vi "Write in Paquetes.vi"(8 "error in (no error)":errorcluster, 11 "TestCase in":refnum<class "Test DataBase.lvclass">) -> (0 "error out":errorcluster, 3 "TestCase out":refnum<class "Test DataBase.lvclass">)   [LabVIEW 2020, in "Test DataBase.lvclass"]
uses:
  Test DataBase.lvclass
  Paquetes Disponibles/Paquetes Disponibles.lvclass
  Paquetes Disponibles/Paquetes Disponibles.lvclass/Paquetes Disponibles.ctl
  <vilib>/addons/_JKI Toolkits/VI Tester/TestCase.llb/TestCase.lvclass
  C:/Program Files (x86)/National Instruments/LabVIEW 2020/vi.lib/addons/_JKI Toolkits/VI Tester/TestCase.llb/TestCase.lvclass
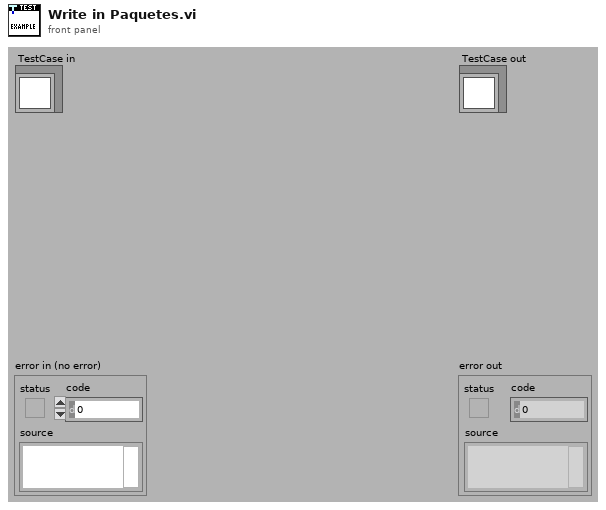
[diagram p1: front panel]
types:
  T1 = cluster{"Name":string, "Cost":u8, "Comprar":bool}[][]
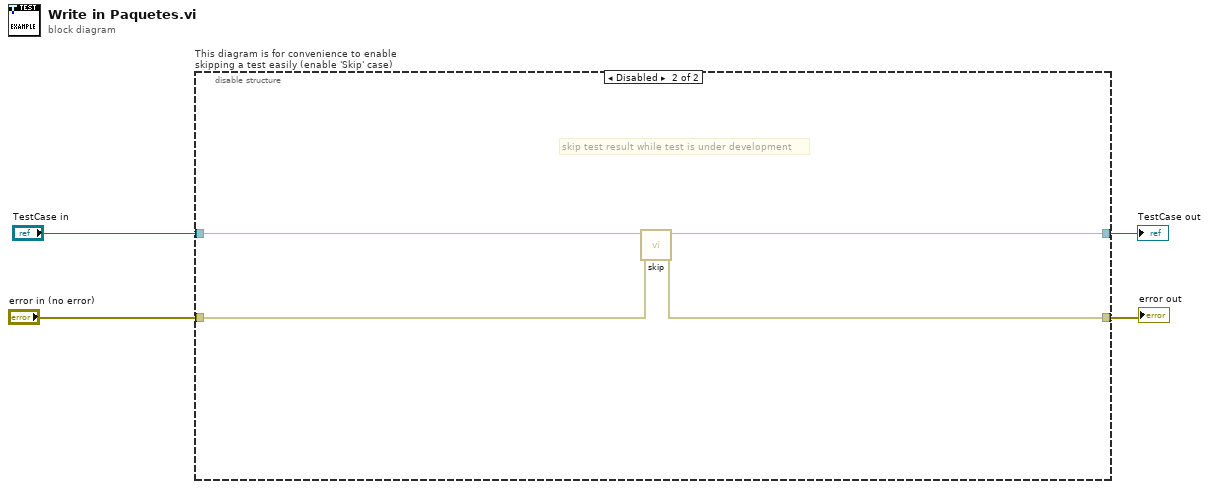
[diagram p0: block diagram]
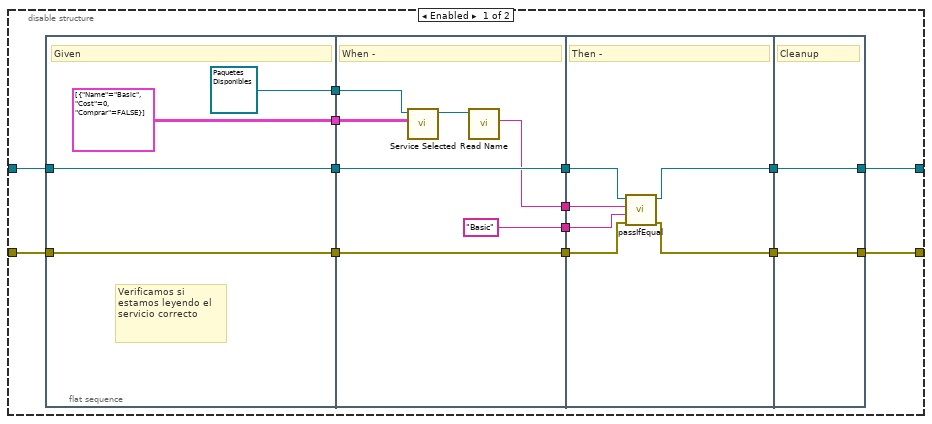
[diagram p2: hidden frame]
diagram:
  n1 = disable-structure "This diagram is for convenience to enable skipping a test easily (enable 'Skip' case)" shown="Disabled" {
    disable-tunnel: "TestCase in" -> [w12 w41]
    disable-tunnel: [w10 w39] -> w1
    disable-tunnel: [w9 w40] -> w3
    disable-tunnel: "error in (no error)" -> [w11 w38]
    frame Enabled {
      n2 = flat-sequence {
        tunnel: w11 -> [w21]
        tunnel: w12 -> [w22]
        tunnel: [w22] -> w18
        tunnel: [w21] -> w17
        tunnel: [refnum<class "Paquetes Disponibles.lvclass"> refnum ("Paquetes Disponibles.lvlib:Paquetes Disponibles.lvclass")] -> w8
        tunnel: [T1 [[{"Name"="Basic", "Cost"=0, "Comprar"=FALSE}]] ("Wash Car Cost")] -> w7
        tunnel: [w29] -> w16
        tunnel: [w28] -> w15
        tunnel: w18 -> [w29]
        tunnel: w17 -> [w28]
        tunnel: w8 -> [w27]
        tunnel: w7 -> [w26]
        tunnel: [w24] -> w6
        tunnel: ["Basic"] -> w5
        tunnel: [w34] -> w14
        tunnel: [w32] -> w13
        tunnel: w16 -> [w35]
        tunnel: w15 -> [w33]
        tunnel: w6 -> [w31]
        tunnel: w5 -> [w30]
        tunnel: [w36] -> w9
        tunnel: [w37] -> w10
        tunnel: w14 -> [w37]
        tunnel: w13 -> [w36]
        frame #0 {
          # "Verificamos si estamos leyendo el servicio correcto"
          # "Given"
        }
        frame #1 {
          # "When -"
          n3 = call "Service Selected.vi"("Wash Car Cost"=w26, "Paquetes Disponibles in"=w27) -> ("Paquetes Disponibles out"=w25:refnum<class "Paquetes Disponibles.lvclass">)  [unwired: 8 in, 1 out]
          n4 = call "Read Name.vi"("Paquetes Disponibles in"=w25) -> ("Name"=w24:string)  [unwired: 8 in, 2 out]
        }
        frame #2 {
          # "Then -"
          n5 = call-dynamic "passIfEqual.vi"("error in (no error)"=w33, "y"=w30, "x"=w31, "TestCase in"=w35) -> ("error out"=w32:errorcluster, "TestCase out"=w34:refnum<class "Test DataBase.lvclass">)  [unwired: 6 in]
        }
        frame #3 {
          # "Cleanup"
        }
      }
    }
    frame Disabled {
      # "skip test result while test is under development"
      n6 = call <vilib>:"skip.vi"("error in (no error)"=w38, "TestCase in"=w41) -> ("error out"=w40:errorcluster, "TestCase out"=w39:refnum<class "Test DataBase.lvclass">)  [unwired: 8 in]
    }
  }
  "error out" <- w3
  "TestCase out" <- w1
